vi "open.vi"(8 "error in (no error)":errorcluster, 9 "Manipulator group (0)":i16, 10 "Timeout (ms) (100)":u16=100, 11 "UDP target address (169.254.255.255)":string="169.254.255.255") -> (0 "error out":errorcluster, 3 "Handle out":i64)   [LabVIEW 2016, in "OSB_uMp_library.lvlib"]
doc: "Open connection to uMp hub/controller"
uses:
  OSB_uMp_library.lvlib
  ump.dll
panel:
  # "By Stuart Box at OxSyBio Ltd, 2017\n\nThis software is provided WITHOUT ANY WARRANTY; without even the implied warranty of MERCHANTABILITY or FITNESS FOR A PARTICULAR PURPOSE.\n\ninfo@oxsybio.com\n\nOxSyBio Ltd, The Walbrook Building, 25 Walbrook, London, EC4N 8AF"
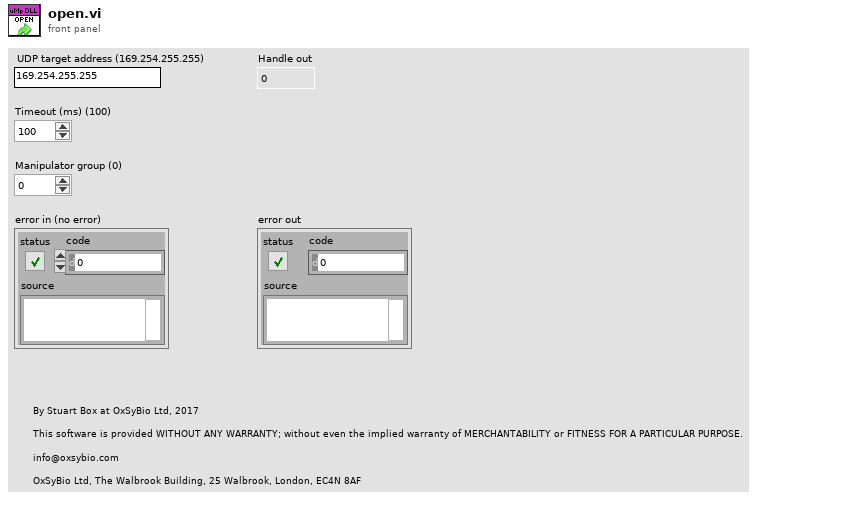
[diagram p1: front panel]
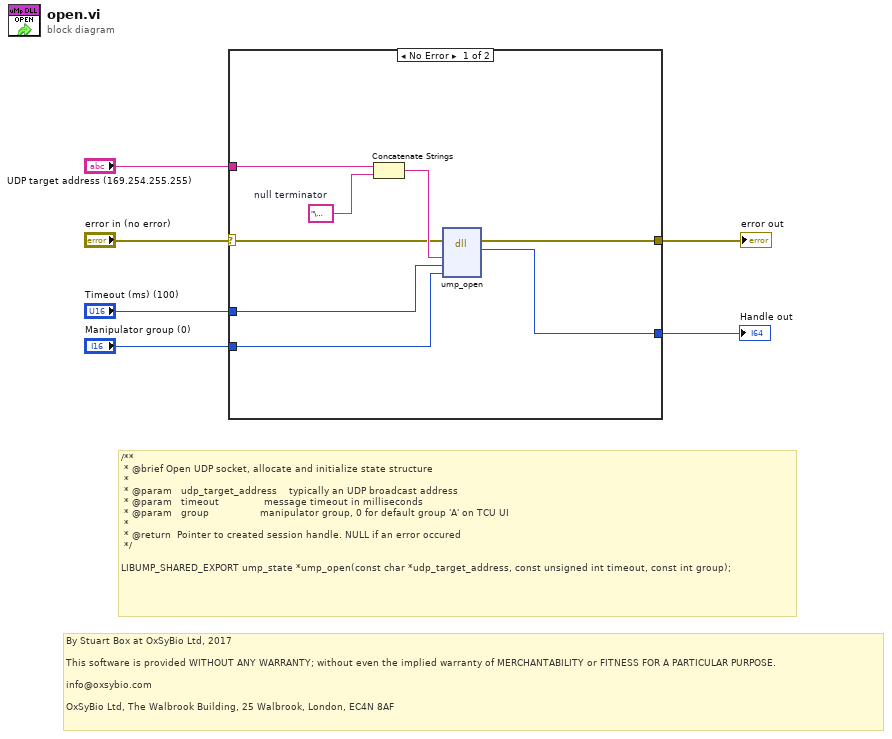
[diagram p0: block diagram]
diagram:
  # "By Stuart Box at OxSyBio Ltd, 2017\n\nThis software is provided WITHOUT ANY WARRANTY; without even the implied warranty of MERCHANTABILITY or FITNESS FOR A PARTICULAR PURPOSE.\n\ninfo@oxsybio.com\n\nOxSyBio Ltd, The Walbrook Building, 25 Walbrook, London, EC4N 8AF"
  # "/**\n * @brief Open UDP socket, allocate and initialize state structure\n *\n * @param   udp_target_address    typically an UDP broadcast address\n * @param   timeout               message timeout in milliseconds\n * @param   group                 manipulator group, 0 for default group 'A' on TCU UI\n *\n * @return  Pointer to created session handle. NULL if an error occured\n */\n\nLIBUMP_SHARED_EXPORT ump_state *ump_open(const char *udp_target_address, const unsigned int timeout, const int group);"
  n1 = case shown="No Error" "error in (no error)" {
    selector: "error in (no error)" -> [w7 w15]
    tunnel: [w14 _] -> w6
    tunnel: [w13 w15] -> w5
    tunnel: "UDP target address (169.254.255.255)" -> [w12 _]
    tunnel: "Timeout (ms) (100)" -> [w9 _]
    tunnel: "Manipulator group (0)" -> [w8 _]
    frame No Error {
      w10 = "\u0000"  # null terminator
      n2 = Concatenate Strings(w12, w10) -> (w11:string)
      n3 = dll-call lib="C:/Users/Stu/Desktop/OSB LabVIEW uMp/uMp_library/ump.dll" fn="ump_open"(error in=w7, "udp_target_address"=w11, "timeout"=w9, "group"=w8) -> (error out=w13:errorcluster, "handle"=w14:i64)  [unwired: 5 in, 1 out]
    }
    frame Error {
    }
  }
  "Handle out" <- w6
  "error out" <- w5
